vi "dead_zone.vi"(1 "min":dbl, 2 "max":dbl, 3 "number in":dbl) -> (0 "number out":dbl)   [LabVIEW 2014]
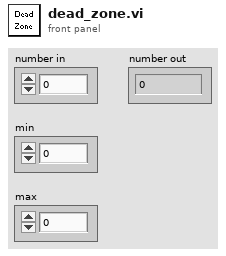
[diagram p1: front panel]
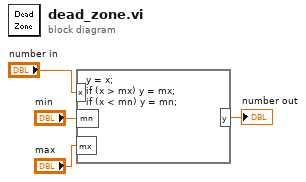
[diagram p0: block diagram]
diagram:
  n1 = formula code="y = x;\nif (x > mx) y = mx;\nif (x < mn) y = mn;"("x"="number in", "mn"="min", "mx"="max") -> ("y"=→"number out":dbl)
